vi "WPI_DashboardProcessTCPPacket.vi"(11 "data in":string) -> (1 "New Robot IP":bool, 2 "Docked":bool, 3 "Robot IP":string, 4 "Power and Errors":T1, 5 "Simulated":bool)   [LabVIEW 2017]
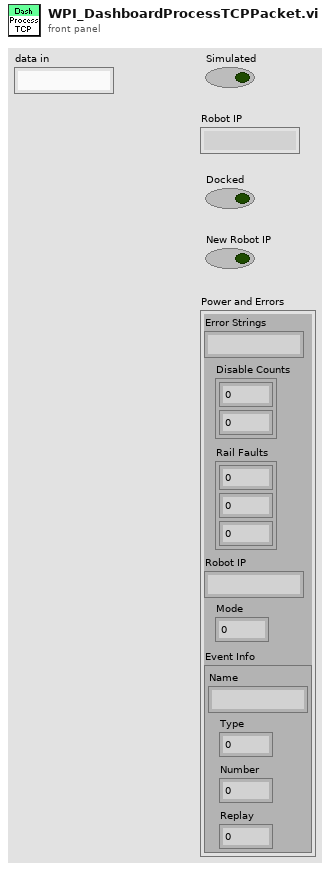
[diagram p1: front panel]
types:
  T1 = cluster{"Error Strings":string, "Disable Counts":cluster{u16, u16}, "Rail Faults":cluster{u16, u16, u16}, "Robot IP":string, "Mode":u8, "Event Info":cluster{"Name":string, "Type":u8, "Number":u16, "Replay":u8}}
  T2 = cluster{"Error Strings":string, "Disable Counts":cluster{u16, u16}, "Rail Faults":cluster{u16, u16, u16}, "Robot IP":string, "Mode":u8, "Event Info":cluster{"Name":string, "Type":u8, "Number":u16, "Replay":u8}, "New Robot IP":bool}
  T3 = cluster{"Name":string, "Type":u8, "Number":u16, "Replay":u8}
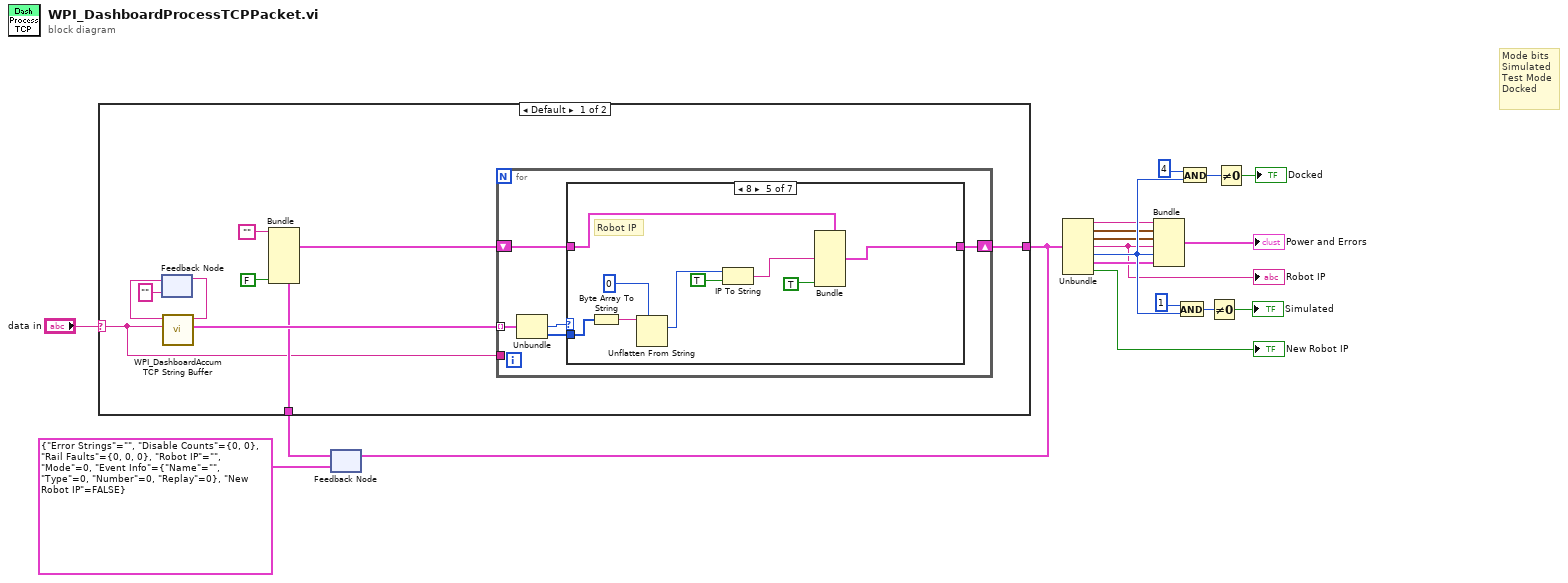
[diagram p0: block diagram]
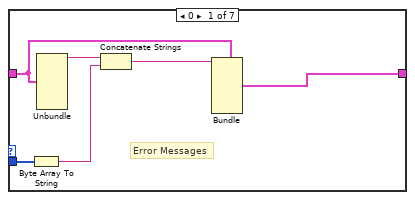
[diagram p2: hidden frame]
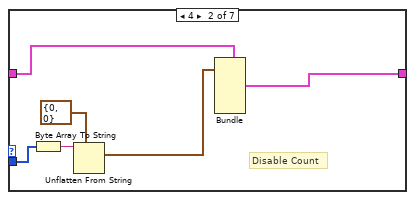
[diagram p3: hidden frame]
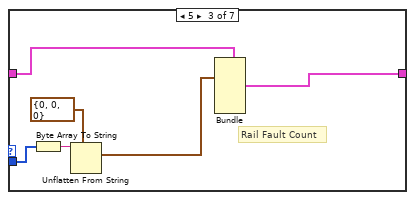
[diagram p4: hidden frame]
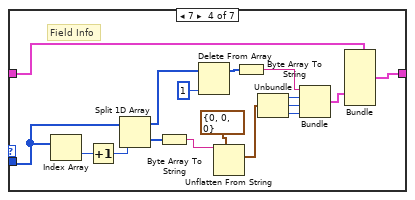
[diagram p5: hidden frame]
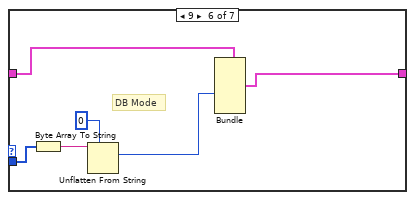
[diagram p6: hidden frame]
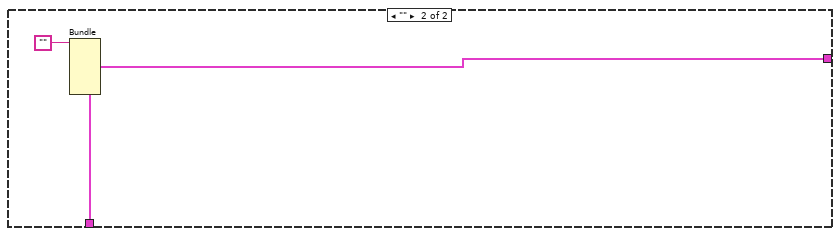
[diagram p8: hidden frame]
diagram:
  # "Mode bits\nSimulated\nTest Mode\nDocked"
  n1 = feedback #1(T2 {"Error Strings"="", "Disable Counts"={0, 0}, "Rail Faults"={0, 0, 0}, "Robot IP"="", "Mode"=0, "Event Info"={"Name"="", "Type"=0, "Number"=0, "Replay"=0}, "New Robot IP"=FALSE} ("Robot Info")) -> (w2:T2)
  n2 = case shown="Default" "data in" {
    selector: "data in" -> [w20 _]
    tunnel: [w24 w87] -> w10
    tunnel: w2 -> [w22 w86]
    frame Default {
      n3 = feedback #2("" ("string")) -> (w27:string)
      n4 = call <vilib>:"WPI_DashboardAccum TCP String Buffer.vi"("data in"=w20, "string in"=w27) -> ("Array"=w25:cluster{u16, u8, "unsigned byte array":u8[]}[], "string out"=w26:string)  [unwired: 8 in]
      n5 = feedback-in #2(w26) -> ()
      n6 = Bundle(cluster=w22, "Error Strings"="", "New Robot IP"=FALSE) -> (w21:T2)  [unwired: 5 in]
      n7 = for {
        tunnel: w25 -> [w31] mode=indexing
        shift-right: [w29] -> w24
        shift-left: w21 -> [w30]
        tunnel: w20 -> [_]
        n8 = Unbundle(w31) -> (w33:u8, "unsigned byte array"=w32:u8[])  [unwired: 1 out]
        n9 = case shown="8" w33 {
          tunnel: w32 -> [w39 w45 w51 w64 w77 w83 _]
          tunnel: w30 -> [w38 w43 w49 w68 w76 w82 w84]
          tunnel: [w34 w42 w48 w67 w75 w81 w84] -> w29
          frame 0 {
            # "Error Messages"
            n10 = Byte Array To String(unsigned byte array=w39) -> (string=w36:string)
            n11 = Unbundle(w38) -> ("Error Strings"=w37:string)  [unwired: 6 out]
            n12 = Concatenate Strings(w37, w36) -> (w35:string)
            n13 = Bundle(cluster=w38, "Error Strings"=w35) -> (w34:T2)  [unwired: 6 in]
          }
          frame 4 {
            # "Disable Count"
            n14 = Byte Array To String(unsigned byte array=w45) -> (string=w44:string)
            n15 = Unflatten From String(type=cluster{u16, u16} {0, 0}, binary string=w44) -> (value=w40:cluster{u16, u16})  [unwired: 3 in, 2 out]
            n16 = Bundle(cluster=w43, "Disable Counts"=w40) -> (w42:T2)  [unwired: 6 in]
          }
          frame 5 {
            # "Rail Fault Count"
            n17 = Byte Array To String(unsigned byte array=w51) -> (string=w50:string)
            n18 = Unflatten From String(type=cluster{u16, u16, u16} {0, 0, 0}, binary string=w50) -> (value=w46:cluster{u16, u16, u16})  [unwired: 3 in, 2 out]
            n19 = Bundle(cluster=w49, "Rail Faults"=w46) -> (w48:T2)  [unwired: 6 in]
          }
          frame 7 {
            # "Field Info"
            n20 = Index Array(array=w64) -> (element=w66:u8)  [unwired: 1 in]
            n21 = Increment(x=w66) -> (x+1=w65:u8)
            n22 = Split 1D Array(array=w64, index=w65) -> (first subarray=w60:u8[], second subarray=w62:u8[])
            n23 = Byte Array To String(unsigned byte array=w62) -> (string=w61:string)
            n24 = Delete From Array(array=w60, index=1) -> (array with subset deleted=w58:u8[])  [unwired: 1 in, 1 out]
            n25 = Unflatten From String(type=cluster{u8, u16, u8} {0, 0, 0}, binary string=w61) -> (value=w55:cluster{u8, u16, u8})  [unwired: 3 in, 2 out]
            n26 = Byte Array To String(unsigned byte array=w58) -> (string=w57:string)
            n27 = Unbundle(w55) -> (w54:u8, w53:u16, w52:u8)
            n28 = Bundle("string"=w57, w54, w53, w52) -> (w56:cluster{"string":string, u8, u16, u8})  [unwired: 1 in]
            n29 = Bundle(cluster=w68, "Event Info"=w56) -> (w67:T2)  [unwired: 6 in]
          }
          frame 8 {
            # "Robot IP"
            n30 = Byte Array To String(unsigned byte array=w77) -> (string=w74:string)
            n31 = Unflatten From String(type=u32 0, binary string=w74) -> (value=w70:u32)  [unwired: 3 in, 2 out]
            n32 = IP To String(1:TRUE ("dot notation? (F)"), 2:w70) -> (0:w69:string)
            n33 = Bundle(cluster=w76, "Robot IP"=w69, "New Robot IP"=TRUE) -> (w75:T2)  [unwired: 5 in]
          }
          frame 9 {
            # "DB Mode"
            n34 = Byte Array To String(unsigned byte array=w83) -> (string=w79:string)
            n35 = Unflatten From String(type=u8 0, binary string=w79) -> (value=w78:u8)  [unwired: 3 in, 2 out]
            n36 = Bundle(cluster=w82, "Mode"=w78) -> (w81:T2)  [unwired: 6 in]
          }
          frame Default {
          }
        }
      }
    }
    frame "" {
      n37 = Bundle(cluster=w86, "Error Strings"="") -> (w87:T2)  [unwired: 6 in]
    }
  }
  n38 = feedback-in #1(w10) -> ()
  n39 = Unbundle(w10) -> ("Error Strings"=w5:string, "Disable Counts"=w8:cluster{u16, u16}, "Rail Faults"=w7:cluster{u16, u16, u16}, "Robot IP"=w1:string, "Mode"=w17:u8, "Event Info"=w6:T3, "New Robot IP"=→"New Robot IP":bool)
  "Robot IP" <- w1
  n40 = Bundle("Error Strings"=w5, "Disable Counts"=w8, "Rail Faults"=w7, "Robot IP"=w1, "Mode"=w17, "Event Info"=w6) -> (→"Power and Errors":T1)  [unwired: 1 in]
  n41 = And(x=1, y=w17) -> (x .and. y?=w15:i32)
  n42 = And(x=4, y=w17) -> (x .and. y?=w13:i32)
  n43 = Not Equal To 0?(x=w15) -> (x != 0?=→"Simulated":bool)
  n44 = Not Equal To 0?(x=w13) -> (x != 0?=→"Docked":bool)
